vi "Class Name to Class ID.vi"(11 "Class Name":string) -> (3 "Class ID":string)   [LabVIEW 2023]
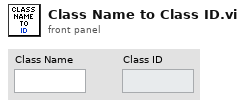
[diagram p1: front panel]
types:
  T1 = cluster{"Class Info":cluster{"Unique ID string":string, "Parent ID string":string, "Class Name (unlocalized)":string, "Class Name (localized)":string}, "Class Heirarchy":string, "Class Type":enum16{"Unknown", "Base", "Scripting", "Private", "Deprecated", "None", "Divider"}, "Indent":u32}[]
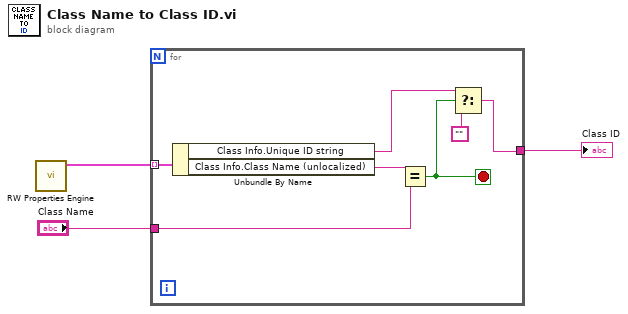
[diagram p0: block diagram]
diagram:
  n1 = call "RW Properties Engine.vi"() -> ("Classes Out"=w3:T1)  [unwired: 6 in, 5 out]
  n2 = for {
    tunnel: w3 -> [w10] mode=indexing
    tunnel: "Class Name" -> [w7]
    tunnel: [w4] -> w1
    stop <- w9 stop-if-true
    n3 = Unbundle By Name(w10) -> ("Class Info.Unique ID string"=w5:string, "Class Info.Class Name (unlocalized)"=w8:string)
    n4 = Equal?(x=w8, y=w7) -> (x = y?=w9:bool)
    n5 = Select(t=w5, s=w9, f="") -> (s? t:f=w4:string)
  }
  "Class ID" <- w1
